vi "FPParseLeidenComputerNames.vi"(8 "error in (no error)":errorcluster, 10 "computer name":string="custardpie") -> (0 "error out":errorcluster, 2 "FP Type":enum32{"CF", "Wet"}(ring))   [LabVIEW 2013]
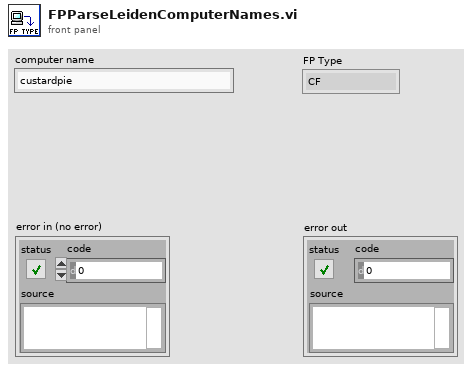
[diagram p1: front panel]
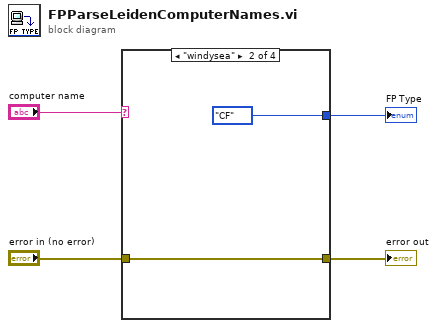
[diagram p0: block diagram]
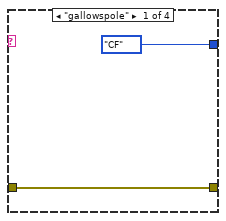
[diagram p2: hidden frame]
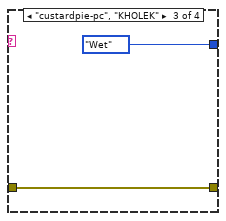
[diagram p3: hidden frame]
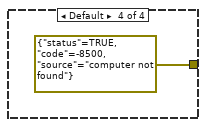
[diagram p4: hidden frame]
diagram:
  n1 = case shown="\"windysea\"" "computer name" {
    tunnel: [enum32{"CF", "Wet"}."CF" ("Type") enum32{"CF", "Wet"}."CF" ("Type") enum32{"CF", "Wet"}."Wet" ("Type") _] -> w4
    tunnel: "error in (no error)" -> [w5 w7 w9 _]
    tunnel: [w5 w7 w9 errorcluster {"status"=TRUE, "code"=-8500, "source"="computer not found"} ("error in (no error)")] -> w1
    frame "gallowspole" {
    }
    frame "windysea" {
    }
    frame "custardpie-pc", "KHOLEK" {
    }
    frame Default {
    }
  }
  "FP Type" <- w4
  "error out" <- w1
